vi "Enqueue Song Requested by UID.vi"(8 "error in (no error)":errorcluster, 10 "UID":string, 11 "MusicManagerActor in":refnum<class "MusicManagerActor.lvclass">) -> (0 "error out":errorcluster, 3 "MusicManagerActor out":refnum<class "MusicManagerActor.lvclass">)   [LabVIEW 2015, in "MusicManagerActor.lvlib" / "MusicManagerActor.lvclass"]
uses:
  MusicManagerActor.lvclass
  MusicManagerActor.lvclass/MusicManagerActor.ctl
  SongQueueActor/SongQueueActor Messages/Add Song To Queue Msg/Add Song To Queue Msg.lvclass
  file/MusicElement/MusicElementLibrary/SongLibrary/SongLibrary.lvclass
  file/MusicElement/Song/Song.lvclass
  file/MusicElement/MusicElementLibrary/MusicLibrary/MusicLibrary.lvclass
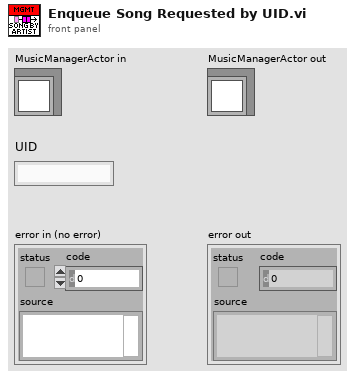
[diagram p1: front panel]
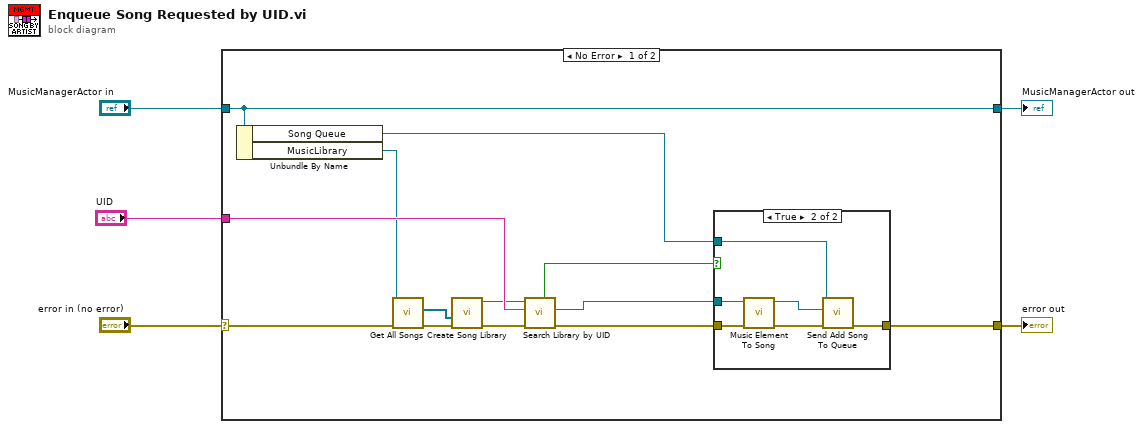
[diagram p0: block diagram]
diagram:
  n1 = case shown="No Error" "error in (no error)" {
    selector: "error in (no error)" -> [w12 w27]
    tunnel: [w17 w27] -> w4
    tunnel: [w18 w26] -> w2
    tunnel: "MusicManagerActor in" -> [w18 w26]
    tunnel: "UID" -> [w15 _]
    frame No Error {
      n2 = Unbundle By Name(w18) -> ("Song Queue"=w16:refnum<class "Message Enqueuer.lvclass">, "MusicLibrary"=w11:refnum<class "MusicLibrary.lvclass">)
      n3 = call "Get All Songs.vi"("error in (no error)"=w12, "MusicLibrary in"=w11) -> ("error out"=w10:errorcluster, "Songs"=w9:refnum<class "Song.lvclass">[])  [unwired: 7 in, 1 out]
      n4 = call "Create Song Library.vi"("error in (no error)"=w10, "Songs"=w9) -> ("error out"=w7:errorcluster, "SongLibrary out"=w8:refnum<class "SongLibrary.lvclass">)  [unwired: 8 in]
      n5 = call "Search Library by UID.vi"("error in (no error)"=w7, "UID"=w15, "SongLibrary"=w8) -> ("error out"=w14:errorcluster, "Song"=w13:refnum<class "Song.lvclass">, "Found?"=w6:bool)  [unwired: 4 in, 2 out]
      n6 = case shown="True" w6 {
        tunnel: [w19 w25] -> w17
        tunnel: w16 -> [_ w24]
        tunnel: w14 -> [w19 w23]
        tunnel: w13 -> [_ w22]
        frame False {
        }
        frame True {
          n7 = call "Music Element To Song.vi"("error in (no error)"=w23, "MusicElement"=w22) -> ("error out"=w21:errorcluster, "Song out"=w20:refnum<class "Song.lvclass">)  [unwired: 8 in]
          n8 = call "Send Add Song To Queue.vi"("error in (no error)"=w21, "Song"=w20, "Message Enqueuer in"=w24) -> ("error out"=w25:errorcluster)  [unwired: 7 in, 1 out]
        }
      }
    }
    frame Error {
    }
  }
  "error out" <- w4
  "MusicManagerActor out" <- w2
